vi "test buffer.vi"() -> ()   [LabVIEW 2018]
panel:
  out "appended array":dbl[](array[numeric])
  out "Array":dbl[](array[numeric])
  in  "stop":bool
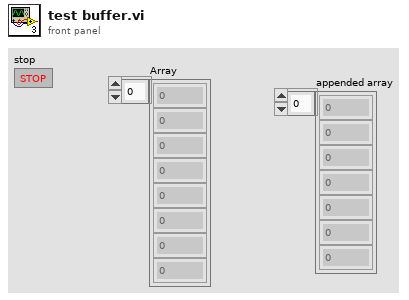
[diagram p1: front panel]
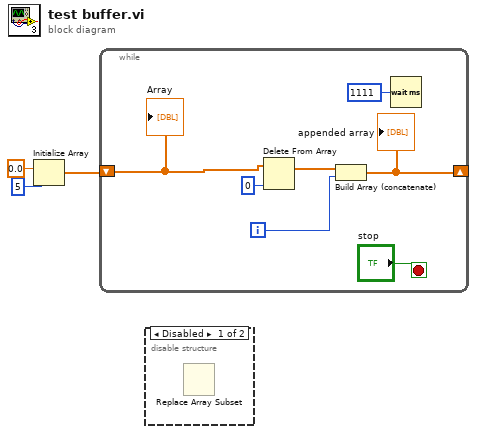
[diagram p0: block diagram]
diagram:
  n1 = Initialize Array(0.0 ("element"), 5 ("dimension size")) -> (w1:dbl[])
  n2 = while {
    shift-right: [w9] -> _
    shift-left: w1 -> [w7]
    i -> [w4]
    stop <- "stop" stop-if-true
    n3 = Delete From Array(array=w7, index=0) -> (array with subset deleted=w5:dbl[])  [unwired: 1 in, 1 out]
    n4 = Build Array (concatenate)(w5, w4) -> (w9:dbl[])
    "appended array" <- w9
    n5 = Wait (ms)(milliseconds to wait=u32 1111) -> ()  [unwired: 1 out]
    "Array" <- w7
  }
  n6 = disable-structure shown="Disabled" {
    frame Disabled {
      n7 = Replace Array Subset() -> ()  [unwired: 3 in, 1 out]
    }
    frame Enabled {
    }
  }
